vi "Calculate Number of Input Samples.vi"(1 "Output Waveform":waveform(dbl)) -> (0 "Number Of Samples":i32)   [LabVIEW 2013]
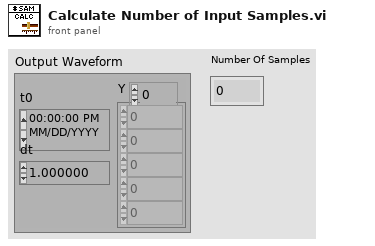
[diagram p1: front panel]
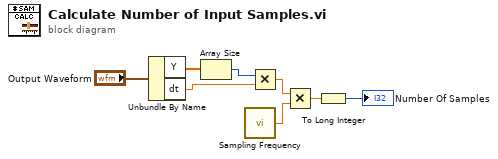
[diagram p0: block diagram]
diagram:
  n1 = Unbundle By Name("Output Waveform") -> ("Y"=w7:dbl[], "dt"=w5:dbl)
  n2 = Array Size(array=w7) -> (size(s)=w6:i32)
  n3 = call "Sampling Frequency.vi"() -> ("Sampling Frequency"=w3:dbl)
  n4 = Multiply(x=w6, y=w5) -> (x*y=w4:dbl)
  n5 = Multiply(x=w4, y=w3) -> (x*y=w2:dbl)
  n6 = To Long Integer(number=w2) -> (32bit integer=→"Number Of Samples":i32)
